vi "Get Dev Product Type.vi"(8 "error in (no error)":errorcluster, 11 "Refnum in":refnum<k21>) -> (0 "error out":errorcluster, 1 "DAQ Type":T1, 2 "ActiveDev":tag, 3 "Refnum out":refnum<k21>)   [LabVIEW 2016, in "Instrument.Lockin.lvclass"]
uses:
  Instrument.Lockin.lvclass
  Typedefs/DAQType-enum.ctl
  <resource>/objmgr/daqmx.rc
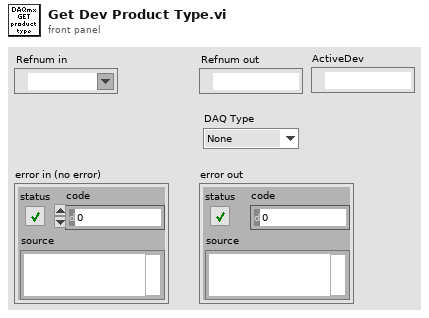
[diagram p1: front panel]
types:
  T1 = typedef "Instrument.Lockin.lvclass/DAQType-enum.ctl" = enum16{"None", "USB 4431", "PXI 446x"}
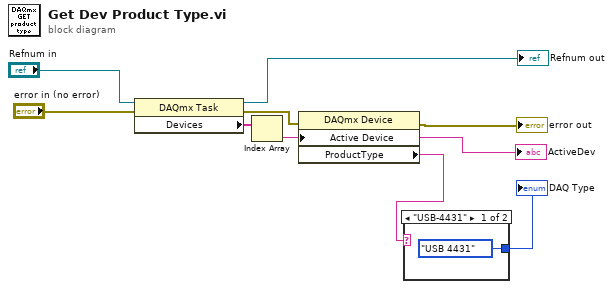
[diagram p0: block diagram]
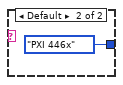
[diagram p2: hidden frame]
diagram:
  n1 = property class="DAQmx Task"(reference="Refnum in", error in="error in (no error)") -> (reference out=→"Refnum out":refnum<k21>, error out=w8:errorcluster, "Devices"=w6:tag[])
  n2 = Index Array(array=w6) -> (element=w3:tag)  [unwired: 1 in]
  "ActiveDev" <- w3
  n3 = property class="DAQmx Device"(error in=w8, "Active Device"=w3) -> (error out=→"error out":errorcluster, "ProductType"=w2:string)  [unwired: 1 in, 1 out]
  n4 = case shown="\"USB-4431\"" w2 {
    tunnel: [DAQType-enum."USB 4431" ("DAQ Type") DAQType-enum."PXI 446x" ("DAQ Type")] -> w1
    frame "USB-4431" {
    }
    frame Default {
    }
  }
  "DAQ Type" <- w1
